vi "mac_mem_dot_product2.vi"() -> ()   [LabVIEW 2014]
uses:
  <vilib>/rvi/XilinxIP/XIPIN_XNode/niFpgaXIPIN.xnode
  <vilib>/Platform/TimedLoop/XDataNode/XDataNode.xnode
  <vilib>/Platform/TimedLoop/XDataNode/nitl_modes.ctl
  <vilib>/Platform/TimedLoop/XDataNode/XDNodeRunTimeDep.lvlib
  <vilib>/Platform/TimedLoop/XDataNode/wakeup.ctl
  <vilib>/Platform/TimedLoop/XDataNode/timing_clust.ctl
  <vilib>/rvi/DataTransferAndStorage/Container/XNode/niFpgaContainer.xnode
  <vilib>/rvi/IPIntegrationNode/IPINode_Xnode/niFpgaIPINode.xnode
  <vilib>/rvi/Memory/Memory_Emulation/niFpgaMemoryEmulationRefIn.vi
  afm_MPC_project/fpga_quadProg/mac_example/Multiply Accumulator12/Multiply_Accumulator12_8251C0362ABC46F4A5B5600C6E330BA5.dll
  MAC_project/mac_example/Multiply Accumulator 6 2 1 2/Multiply_Accumulator_6_2_1_2_02FD3C74846A4C02A23212CAACE05444.dll
  afm_MPC_project/fpga_quadProg/mac_example/Multiply Accumulator10/Multiply_Accumulator10_12FF9FB1410E45B083B4D52CE0C0E68A.dll
  afm_MPC_project/fpga_quadProg/mac_example/Multiply Accumulator09/Multiply_Accumulator09_5D60E3E552CB475F9C9DEB2CB9D60D9C.dll
  afm_MPC_project/fpga_quadProg/mac_example/Multiply Accumulator08/Multiply_Accumulator08_63B3B19177EB4E2C93FF5B78B22982AF.dll
  afm_MPC_project/fpga_quadProg/mac_example/Multiply Accumulator07/Multiply_Accumulator07_E764427B2AF0450BAE442029304CE909.dll
  afm_MPC_project/fpga_quadProg/mac_example/Multiply Accumulator05/Multiply_Accumulator05_30F34FE4A0744937816A99E0FF75C50A.dll
  afm_MPC_project/fpga_quadProg/mac_example/Multiply Accumulator04/Multiply_Accumulator04_4CB6AC15FF37476DBC15807E3D8215EA.dll
  afm_MPC_project/fpga_quadProg/mac_example/Multiply Accumulator03/Multiply_Accumulator03_801B681484E74D9B98E4BDB409AD9BD2.dll
  afm_MPC_project/fpga_quadProg/mac_example/Multiply Accumulator02/Multiply_Accumulator02_E9BD86879A6F4953AE28C6201495FEE1.dll
  afm_MPC_project/fpga_quadProg/mac_example/Multiply Accumulator01/Multiply_Accumulator01_75DB40A42D7149569D987152CB0D01C1.dll
  afm_MPC_project/fpga_quadProg/mac_example/Multiply Accumulator13/Multiply_Accumulator13_12AB7DA088AB48F383581A6BB4F5EF48.dll
  afm_MPC_project/fpga_quadProg/mac_example/Multiply Accumulator15/Multiply_Accumulator15_AA46839E45CE4F01941F3EA3B8C129F7.dll
  afm_MPC_project/fpga_quadProg/mac_example/Multiply Accumulator16/Multiply_Accumulator16_19D64967FE2446C38501744F7FD46696.dll
  afm_MPC_project/fpga_quadProg/mac_example/Multiply Accumulator17/Multiply_Accumulator17_68B37788AA734A29A986F77D953AD864.dll
  afm_MPC_project/fpga_quadProg/mac_example/Multiply Accumulator18/Multiply_Accumulator18_9000D848DA044E598463B90A0F5FDA52.dll
  afm_MPC_project/fpga_quadProg/mac_example/Multiply Accumulator19/Multiply_Accumulator19_D9569D38672A42FAB612A6C6146A7F7D.dll
  afm_MPC_project/fpga_quadProg/mac_example/Multiply Accumulator20/Multiply_Accumulator20_39D8BFFDA167413996EF3D9E83AB1150.dll
  afm_MPC_project/fpga_quadProg/mac_example/Multiply Accumulator21/Multiply_Accumulator21_1E0469235E034C438B32764042598187.dll
  afm_MPC_project/fpga_quadProg/mac_example/Multiply Accumulator22/Multiply_Accumulator22_BD44292DDFE84C49BBDF0A5781548576.dll
  afm_MPC_project/fpga_quadProg/mac_example/Multiply Accumulator23/Multiply_Accumulator23_14E7B3DBE11448D3B90B25377FD6EA57.dll
  afm_MPC_project/fpga_quadProg/mac_example/Multiply Accumulator24/Multiply_Accumulator24_B8B0017A331E415CA2A56A1A38052C9D.dll
  MAC_project/mac_example/Multiply Accumulator06 2/Multiply_Accumulator06_2_FA45EE958C1E4FC79E4A67AB6AD01B1E.dll
  afm_MPC_project/fpga_quadProg/mac_example/Multiply Accumulator14/Multiply_Accumulator14_5D647B84DE964E6297114951802A7EF8.dll
  <vilib>/rvi/IPIntegrationNode/IPINode_Typedef/niFpgaIPINodeSupportedFamilies.ctl
  <vilib>/rvi/IPIntegrationNode/IPINode_Utilities/niFpgaIPINodeSimCore.vi
panel:
  in  "Ns":i16
  out "appended array":fxp<+/-,32,7>[](array[numeric])
  out "s":fxp<+/-,32,7>
  in  "Array":fxp<+/-,18,5>[](array[numeric])=[0.0, 0.0, 0.0, 0.0, 0.0, 0.0, 0.0, 0.0, 0.0, 0.0, 0.0, 0.0, 0.0, 0.0, 0.0, 0.0, 0.0, 0.0, 0.0, 0.0, 0.0, 0.0, 0.0, 0.0]
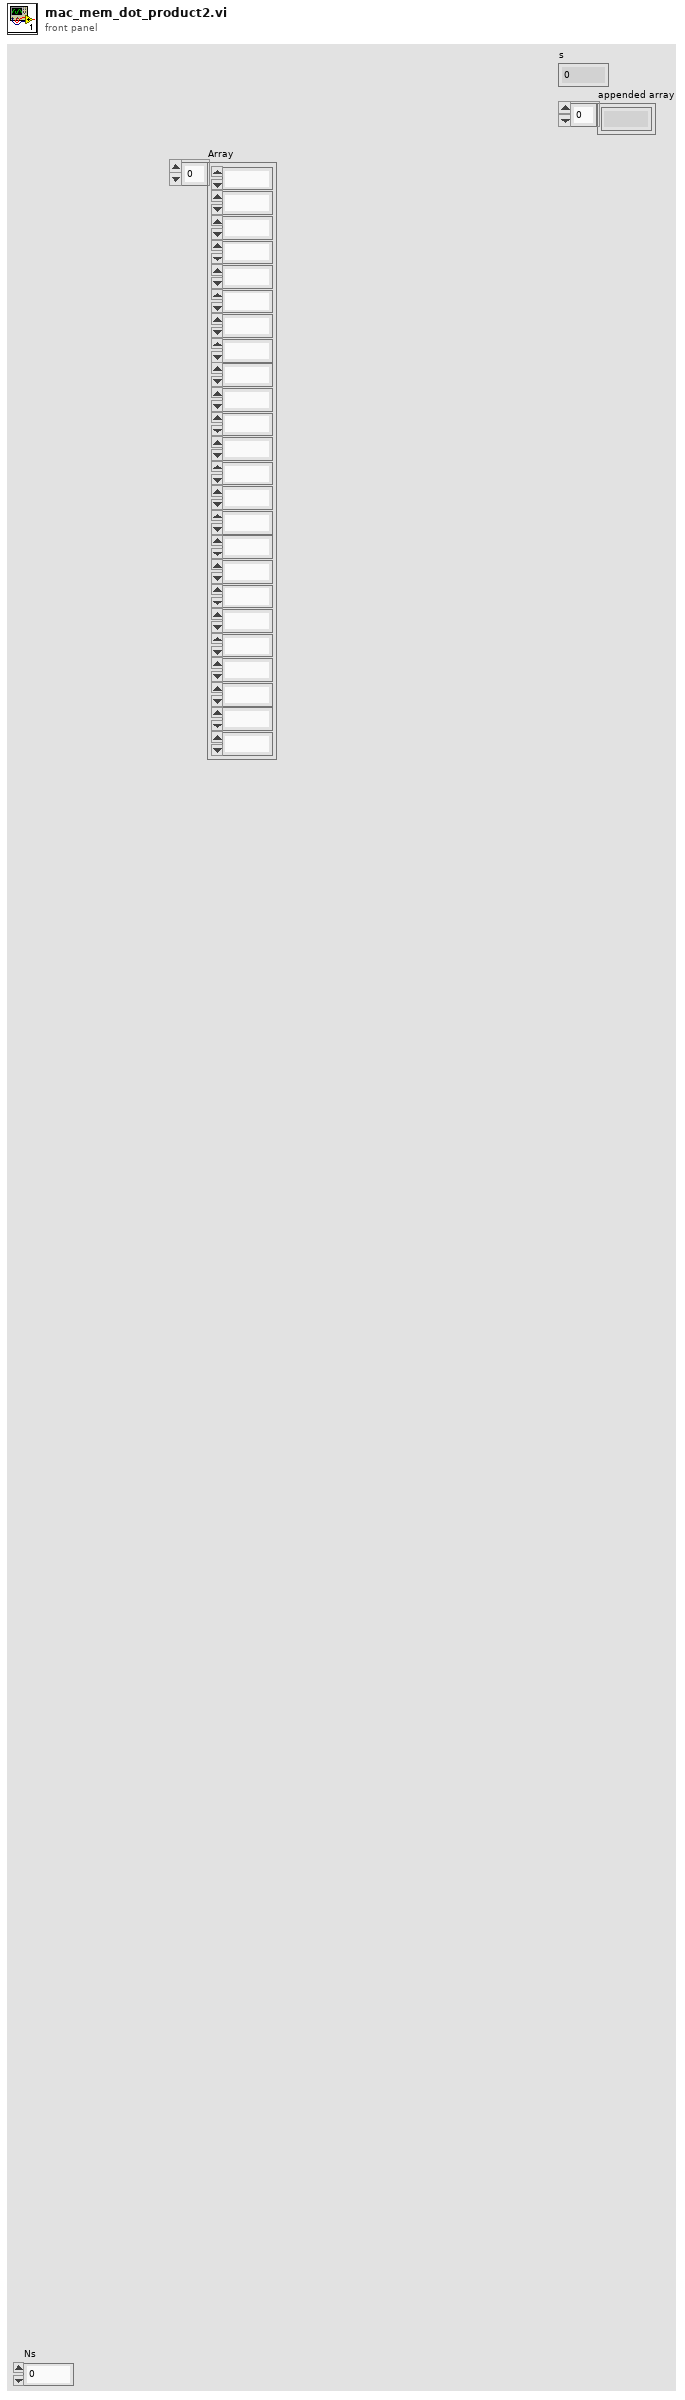
[diagram p1: front panel]
types:
  T1 = typedef "XDNodeRunTimeDep.lvlib/timing_clust.ctl" = cluster{"Expected End [f-1]":u64, "Actual End [f-1]":u64, "Finished Late? [f-1]":bool, "Expected End [i-1]":u64, "Actual End [i-1]":u64, "Finished Late? [i-1]":bool, "Expected Start [i]":u64, "Actual Start [i]":u64, "Expected Start [f]":u64, "Actual Start [f]":u64, "Source Name":string, "Structure Name":string, "Period":i64, "Deadline":i64, "Offset":i64, "Start":i64, "Priority":i32, "Timeout":i32, "Mode":T2, "Wakeup Reason":T3, "Error":errorcluster, "Source Type":string, "Secondary Source Type":string, "Global End Time":u64, "Global Start Time":u64, "Frame Duration":u64, "Iteration Duration":u64, "Assigned CPU":i32, "I/O Scan Engine Mode":u32}
  T2 = typedef "XDNodeRunTimeDep.lvlib/nitl_modes.ctl" = enum32{"No Change", "Process missed periods, maintain original phase", "Discard missed periods, maintain original phase", "Process missed periods, ignore original phase", "Discard missed periods, ignore original phase"}
  T3 = typedef "XDNodeRunTimeDep.lvlib/wakeup.ctl" = enum32{"Normal", "Aborted", "Asynchronous wakeup", "Timing source error", "Timed loop error", "Timeout"}
  T4 = typedef "niFpgaIPINodeSupportedFamilies.ctl" = cluster{"unlimited?":bool, "supported targets":string[]}
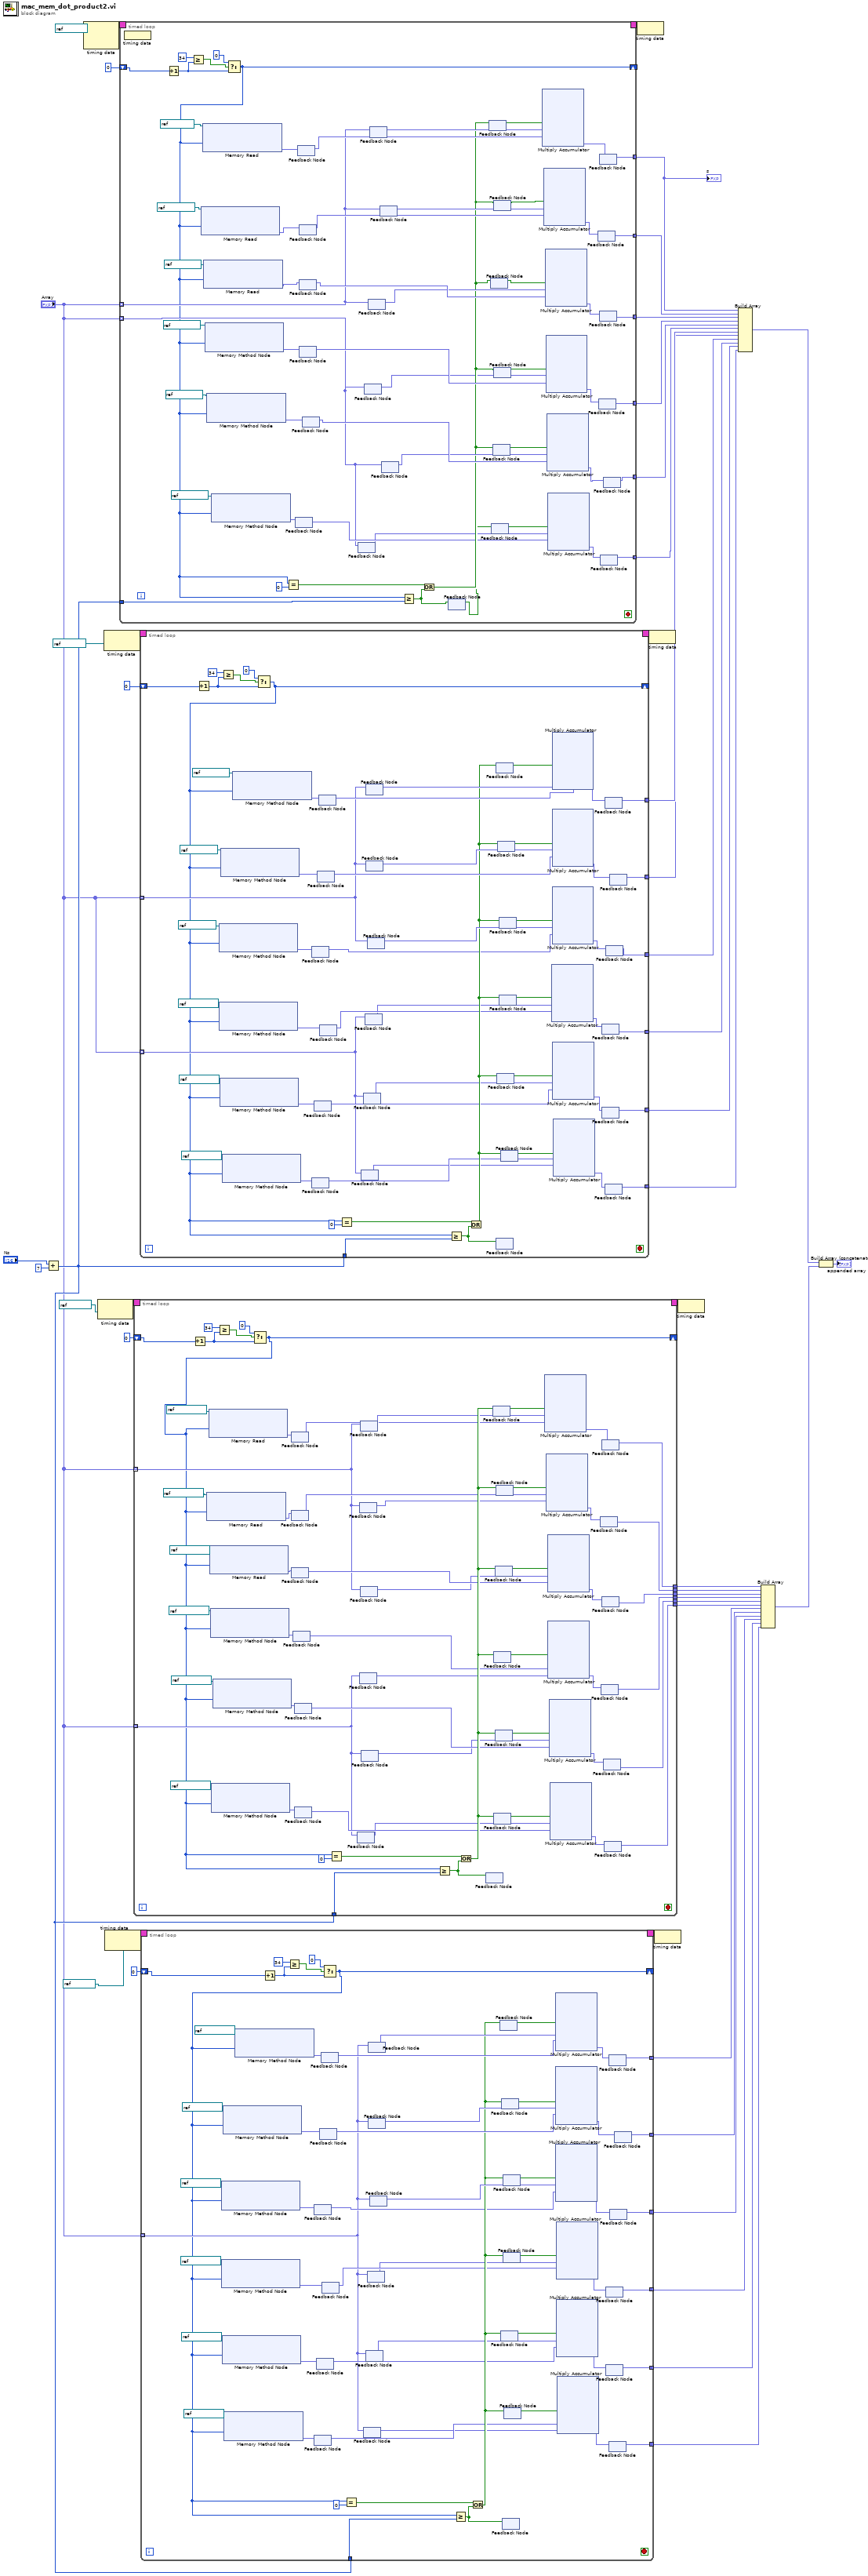
[diagram p0: block diagram]
diagram:
  n1 = Add(x="Ns", y=i16 7) -> (x+y=w8:i16)
  n2 = node-c288(refnum<k21> "160MHz" ("Source Name")) -> (w21:T1)  [unwired: 1 in]
  n3 = node-c288(refnum<k21> "160MHz" ("Source Name")) -> (w13:T1)
  n4 = node-c288(refnum<k21> "160MHz" ("Source Name")) -> (w19:T1)
  n5 = node-c288(refnum<k21> "160MHz" ("Source Name")) -> (w10:T1)
  n6 = timed-loop {
    timing: w21 -> [_]
    timing-out: [_] -> w20
    tunnel: [w103] -> w47
    tunnel: [w102] -> w46
    tunnel: [w101] -> w45
    tunnel: [w100] -> w44
    tunnel: [w99] -> w43
    tunnel: "Array" -> [w64] mode=indexing
    tunnel: w8 -> [w85]
    tunnel: "Array" -> [w56] mode=indexing
    tunnel: [w55] -> w6
    shift-right: [w48] -> _
    shift-left: i16 0 -> [w53]
    stop <- _ stop-if-true
    n7 = node-c288() -> ()  [unwired: 1 in]
    n8 = Increment(x=w53) -> (x+1=w52:i16)
    n9 = Greater Or Equal?(x=i16 34, y=w52) -> (x >= y?=w51:bool)
    n10 = Select(t=i16 0, s=w51, f=w52) -> (s? t:f=w48:i16)
    n11 = xnode ("Memory Read")("Address"=w48, "Memory In"=refnum<k21> "Memory 2") -> ("Data"=w80:fxp<+/-,32,2>)  [unwired: 1 out]
    n12 = xnode ("Memory Read")("Address"=w48, "Memory In"=refnum<k21> "Memory") -> ("Data"=w84:fxp<+/-,32,2>)  [unwired: 1 out]
    n13 = xnode ("Memory Read")("Address"=w48, "Memory In"=refnum<k21> "Memory 3") -> ("Data"=w77:fxp<+/-,32,2>)  [unwired: 1 out]
    n14 = xnode ("Memory Method Node")("Address"=w48, "Memory In"=refnum<k21> "Memory 4") -> ("Data"=w74:fxp<+/-,32,2>)  [unwired: 1 out]
    n15 = xnode ("Memory Method Node")("Address"=w48, "Memory In"=refnum<k21> "Memory 5") -> ("Data"=w72:fxp<+/-,32,2>)  [unwired: 1 out]
    n16 = xnode ("Memory Method Node")("Address"=w48, "Memory In"=refnum<k21> "Memory 6") -> ("Data"=w62:fxp<+/-,32,2>)  [unwired: 1 out]
    n17 = Equal?(x=w48, y=0) -> (x = y?=w86:bool)
    n18 = feedback #1() -> (w59:fxp<+/-,32,2>)  [unwired: 1 in]
    n19 = feedback-in #1(w62) -> ()
    n20 = feedback #2() -> (w83:fxp<+/-,32,2>)  [unwired: 1 in]
    n21 = feedback-in #2(w84) -> ()
    n22 = feedback #3() -> (w81:fxp<+/-,32,2>)  [unwired: 1 in]
    n23 = feedback-in #3(w80) -> ()
    n24 = feedback #4() -> (w78:fxp<+/-,32,2>)  [unwired: 1 in]
    n25 = feedback-in #4(w77) -> ()
    n26 = feedback #5() -> (w75:fxp<+/-,32,2>)  [unwired: 1 in]
    n27 = feedback-in #5(w74) -> ()
    n28 = feedback #6() -> (w73:fxp<+/-,32,2>)  [unwired: 1 in]
    n29 = feedback-in #6(w72) -> ()
    n30 = feedback #7() -> (w58:fxp<+/-,18,5>)  [unwired: 1 in]
    n31 = feedback-in #7(w56) -> ()
    n32 = feedback #8() -> (w54:fxp<+/-,18,5>)  [unwired: 1 in]
    n33 = feedback-in #8(w56) -> ()
    n34 = feedback #9() -> (w76:fxp<+/-,18,5>)  [unwired: 1 in]
    n35 = feedback-in #9(w64) -> ()
    n36 = feedback #10() -> (w82:fxp<+/-,18,5>)  [unwired: 1 in]
    n37 = feedback-in #10(w64) -> ()
    n38 = feedback #11() -> (w79:fxp<+/-,18,5>)  [unwired: 1 in]
    n39 = feedback-in #11(w64) -> ()
    n40 = feedback #12() -> (w71:fxp<+/-,18,5>)  [unwired: 1 in]
    n41 = feedback-in #12(w56) -> ()
    n42 = Greater Or Equal?(x=w48, y=w85) -> (x >= y?=w70:bool)
    n43 = Or(x=w86, y=w70) -> (x .or. y?=w66:bool)
    n44 = feedback #13() -> (w57:bool)  [unwired: 1 in]
    n45 = feedback-in #13(w70) -> ()
    n46 = feedback #14() -> (w65:bool)  [unwired: 1 in]
    n47 = feedback-in #14(w66) -> ()
    n48 = feedback #15() -> (w68:bool)  [unwired: 1 in]
    n49 = feedback-in #15(w66) -> ()
    n50 = feedback #16() -> (w61:bool)  [unwired: 1 in]
    n51 = feedback-in #16(w57) -> ()
    n52 = feedback #17() -> (w93:bool)  [unwired: 1 in]
    n53 = feedback-in #17(w66) -> ()
    n54 = feedback #18() -> (w69:bool)  [unwired: 1 in]
    n55 = feedback-in #18(w66) -> ()
    n56 = feedback #19() -> (w67:bool)  [unwired: 1 in]
    n57 = feedback-in #19(w66) -> ()
    n58 = xnode ("Multiply Accumulator")("sclr"=w65, "b"=w82, "a"=w83) -> ("s"=w88:fxp<+/-,32,7>)  [unwired: 2 in]
    n59 = xnode ("Multiply Accumulator")("sclr"=w67, "b"=w79, "a"=w81) -> ("s"=w89:fxp<+/-,32,7>)  [unwired: 2 in]
    n60 = xnode ("Multiply Accumulator")("sclr"=w68, "b"=w76, "a"=w78) -> ("s"=w90:fxp<+/-,32,7>)  [unwired: 2 in]
    n61 = xnode ("Multiply Accumulator")("sclr"=w69, "b"=w54, "a"=w75) -> ("s"=w91:fxp<+/-,32,7>)  [unwired: 2 in]
    n62 = xnode ("Multiply Accumulator")("sclr"=w93, "b"=w71, "a"=w73) -> ("s"=w92:fxp<+/-,18,7>)  [unwired: 2 in]
    n63 = xnode ("Multiply Accumulator")("sclr"=w61, "b"=w58, "a"=w59) -> ("s"=w60:fxp<+/-,32,7>)  [unwired: 2 in]
    n64 = feedback #20() -> (w102:fxp<+/-,32,7>)  [unwired: 1 in]
    n65 = feedback-in #20(w89) -> ()
    n66 = feedback #21() -> (w100:fxp<+/-,32,7>)  [unwired: 1 in]
    n67 = feedback-in #21(w91) -> ()
    n68 = feedback #22() -> (w103:fxp<+/-,32,7>)  [unwired: 1 in]
    n69 = feedback-in #22(w88) -> ()
    n70 = feedback #23() -> (w101:fxp<+/-,32,7>)  [unwired: 1 in]
    n71 = feedback-in #23(w90) -> ()
    n72 = feedback #24() -> (w55:fxp<+/-,32,7>)  [unwired: 1 in]
    n73 = feedback-in #24(w60) -> ()
    n74 = feedback #25() -> (w99:fxp<+/-,18,7>)  [unwired: 1 in]
    n75 = feedback-in #25(w92) -> ()
  }
  "s" <- w47
  n76 = timed-loop {
    timing: w13 -> [_]
    timing-out: [_] -> w12
    tunnel: [w439] -> w36
    tunnel: [w438] -> w35
    tunnel: [w437] -> w34
    tunnel: [w436] -> w33
    tunnel: [w435] -> w32
    tunnel: [w434] -> w31
    tunnel: "Array" -> [w392] mode=indexing
    tunnel: w8 -> [w406]
    tunnel: "Array" -> [w391] mode=indexing
    shift-right: [w385] -> _
    shift-left: i16 0 ("t") -> [w386]
    stop <- _ stop-if-true
    n77 = Increment(x=w386) -> (x+1=w390:i16)
    n78 = Greater Or Equal?(x=i16 34, y=w390) -> (x >= y?=w389:bool)
    n79 = Select(t=i16 0, s=w389, f=w390) -> (s? t:f=w385:i16)
    n80 = xnode ("Memory Read")("Address"=w385, "Memory In"=refnum<k21> "Memory 14") -> ("Data"=w431:fxp<+/-,32,2>)  [unwired: 1 out]
    n81 = xnode ("Memory Read")("Address"=w385, "Memory In"=refnum<k21> "Memory 13") -> ("Data"=w430:fxp<+/-,32,2>)  [unwired: 1 out]
    n82 = xnode ("Memory Read")("Address"=w385, "Memory In"=refnum<k21> "Memory 15") -> ("Data"=w428:fxp<+/-,32,2>)  [unwired: 1 out]
    n83 = xnode ("Memory Method Node")("Address"=w385, "Memory In"=refnum<k21> "Memory 16") -> ("Data"=w426:fxp<+/-,32,2>)  [unwired: 1 out]
    n84 = xnode ("Memory Method Node")("Address"=w385, "Memory In"=refnum<k21> "Memory 18") -> ("Data"=w422:fxp<+/-,32,2>)  [unwired: 1 out]
    n85 = xnode ("Memory Method Node")("Address"=w385, "Memory In"=refnum<k21> "Memory 17") -> ("Data"=w424:fxp<+/-,32,2>)  [unwired: 1 out]
    n86 = feedback #26() -> (w401:fxp<+/-,32,2>)  [unwired: 1 in]
    n87 = feedback-in #26(w431) -> ()
    n88 = feedback #27() -> (w403:fxp<+/-,32,2>)  [unwired: 1 in]
    n89 = feedback-in #27(w430) -> ()
    n90 = feedback #28() -> (w400:fxp<+/-,32,2>)  [unwired: 1 in]
    n91 = feedback-in #28(w428) -> ()
    n92 = feedback #29() -> (w398:fxp<+/-,32,2>)  [unwired: 1 in]
    n93 = feedback-in #29(w426) -> ()
    n94 = feedback #30() -> (w396:fxp<+/-,32,2>)  [unwired: 1 in]
    n95 = feedback-in #30(w424) -> ()
    n96 = feedback #31() -> (w394:fxp<+/-,32,2>)  [unwired: 1 in]
    n97 = feedback-in #31(w422) -> ()
    n98 = Equal?(x=w385, y=0) -> (x = y?=w408:bool)
    n99 = feedback #32() -> (w393:fxp<+/-,18,5>)  [unwired: 1 in]
    n100 = feedback-in #32(w391) -> ()
    n101 = feedback #33() -> (w402:fxp<+/-,18,5>)  [unwired: 1 in]
    n102 = feedback-in #33(w392) -> ()
    n103 = feedback #34() -> (w397:fxp<+/-,18,5>)  [unwired: 1 in]
    n104 = feedback-in #34(w391) -> ()
    n105 = feedback #35() -> (w404:fxp<+/-,18,5>)  [unwired: 1 in]
    n106 = feedback-in #35(w392) -> ()
    n107 = feedback #36() -> (w399:fxp<+/-,18,5>)  [unwired: 1 in]
    n108 = feedback-in #36(w392) -> ()
    n109 = feedback #37() -> (w395:fxp<+/-,18,5>)  [unwired: 1 in]
    n110 = feedback-in #37(w391) -> ()
    n111 = Greater Or Equal?(x=w385, y=w406) -> (x >= y?=w407:bool)
    n112 = Or(x=w408, y=w407) -> (x .or. y?=w405:bool)
    n113 = feedback #38() -> ()  [unwired: 2 in]
    n114 = feedback-in #38(w407) -> ()
    n115 = feedback #39() -> (w416:bool)  [unwired: 1 in]
    n116 = feedback-in #39(w405) -> ()
    n117 = feedback #40() -> (w419:bool)  [unwired: 1 in]
    n118 = feedback-in #40(w405) -> ()
    n119 = feedback #41() -> (w421:bool)  [unwired: 1 in]
    n120 = feedback-in #41(w405) -> ()
    n121 = feedback #42() -> (w418:bool)  [unwired: 1 in]
    n122 = feedback-in #42(w405) -> ()
    n123 = feedback #43() -> (w420:bool)  [unwired: 1 in]
    n124 = feedback-in #43(w405) -> ()
    n125 = feedback #44() -> (w417:bool)  [unwired: 1 in]
    n126 = feedback-in #44(w405) -> ()
    n127 = xnode ("Multiply Accumulator")("sclr"=w416, "b"=w404, "a"=w403) -> ("s"=w410:fxp<+/-,32,7>)  [unwired: 2 in]
    n128 = xnode ("Multiply Accumulator")("sclr"=w417, "a"=w401, "b"=w402) -> ("s"=w411:fxp<+,16,16>)  [unwired: 2 in]
    n129 = xnode ("Multiply Accumulator")("sclr"=w418, "b"=w399, "a"=w400) -> ("s"=w412:fxp<+/-,32,7>)  [unwired: 2 in]
    n130 = xnode ("Multiply Accumulator")("sclr"=w419, "b"=w397, "a"=w398) -> ("s"=w413:fxp<+/-,32,7>)  [unwired: 2 in]
    n131 = xnode ("Multiply Accumulator")("sclr"=w420, "b"=w395, "a"=w396) -> ("s"=w414:fxp<+/-,32,7>)  [unwired: 2 in]
    n132 = xnode ("Multiply Accumulator")("sclr"=w421, "b"=w393, "a"=w394) -> ("s"=w415:fxp<+/-,32,7>)  [unwired: 2 in]
    n133 = feedback #45() -> (w438:fxp<+,16,16>)  [unwired: 1 in]
    n134 = feedback-in #45(w411) -> ()
    n135 = feedback #46() -> (w436:fxp<+/-,32,7>)  [unwired: 1 in]
    n136 = feedback-in #46(w413) -> ()
    n137 = feedback #47() -> (w439:fxp<+/-,32,7>)  [unwired: 1 in]
    n138 = feedback-in #47(w410) -> ()
    n139 = feedback #48() -> (w437:fxp<+/-,32,7>)  [unwired: 1 in]
    n140 = feedback-in #48(w412) -> ()
    n141 = feedback #49() -> (w435:fxp<+/-,32,7>)  [unwired: 1 in]
    n142 = feedback-in #49(w414) -> ()
    n143 = feedback #50() -> (w434:fxp<+/-,32,7>)  [unwired: 1 in]
    n144 = feedback-in #50(w415) -> ()
  }
  n145 = timed-loop {
    timing: w19 -> [_]
    timing-out: [_] -> w18
    tunnel: w8 -> [w826]
    tunnel: [w825] -> w42
    tunnel: [w824] -> w41
    tunnel: [w823] -> w40
    tunnel: [w822] -> w39
    tunnel: [w821] -> w38
    tunnel: [w820] -> w37
    tunnel: "Array" -> [w779] mode=indexing
    tunnel: "Array" -> [w778] mode=indexing
    shift-right: [w772] -> _
    shift-left: i16 0 ("t") -> [w773]
    stop <- _ stop-if-true
    n146 = Increment(x=w773) -> (x+1=w777:i16)
    n147 = Greater Or Equal?(x=i16 34, y=w777) -> (x >= y?=w776:bool)
    n148 = Select(t=i16 0, s=w776, f=w777) -> (s? t:f=w772:i16)
    n149 = xnode ("Memory Method Node")("Address"=w772, "Memory In"=refnum<k21> "Memory 9") -> ("Data"=w794:fxp<+/-,32,2>)  [unwired: 1 out]
    n150 = xnode ("Memory Method Node")("Address"=w772, "Memory In"=refnum<k21> "Memory 10") -> ("Data"=w795:fxp<+/-,32,2>)  [unwired: 1 out]
    n151 = xnode ("Memory Method Node")("Address"=w772, "Memory In"=refnum<k21> "Memory 11") -> ("Data"=w796:fxp<+/-,32,2>)  [unwired: 1 out]
    n152 = xnode ("Memory Method Node")("Address"=w772, "Memory In"=refnum<k21> "Memory 8") -> ("Data"=w808:fxp<+/-,32,2>)  [unwired: 1 out]
    n153 = xnode ("Memory Method Node")("Address"=w772, "Memory In"=refnum<k21> "Memory 12") -> ("Data"=w797:fxp<+/-,32,2>)  [unwired: 1 out]
    n154 = xnode ("Memory Method Node")("Address"=w772, "Memory In"=refnum<k21> "Memory 7") -> ("Data"=w806:fxp<+/-,32,2>)  [unwired: 1 out]
    n155 = feedback #51() -> (w793:fxp<+/-,32,2>)  [unwired: 1 in]
    n156 = feedback-in #51(w794) -> ()
    n157 = feedback #52() -> (w790:fxp<+/-,32,2>)  [unwired: 1 in]
    n158 = feedback-in #52(w797) -> ()
    n159 = feedback #53() -> (w791:fxp<+/-,32,2>)  [unwired: 1 in]
    n160 = feedback-in #53(w796) -> ()
    n161 = feedback #54() -> (w807:fxp<+/-,32,2>)  [unwired: 1 in]
    n162 = feedback-in #54(w808) -> ()
    n163 = feedback #55() -> (w805:fxp<+/-,32,2>)  [unwired: 1 in]
    n164 = feedback-in #55(w806) -> ()
    n165 = feedback #56() -> (w792:fxp<+/-,32,2>)  [unwired: 1 in]
    n166 = feedback-in #56(w795) -> ()
    n167 = Equal?(x=w772, y=0) -> (x = y?=w818:bool)
    n168 = feedback #57() -> (w787:fxp<+/-,18,5>)  [unwired: 1 in]
    n169 = feedback-in #57(w778) -> ()
    n170 = feedback #58() -> (w788:fxp<+/-,18,5>)  [unwired: 1 in]
    n171 = feedback-in #58(w778) -> ()
    n172 = feedback #59() -> (w789:fxp<+/-,18,5>)  [unwired: 1 in]
    n173 = feedback-in #59(w778) -> ()
    n174 = feedback #60() -> (w814:fxp<+/-,18,5>)  [unwired: 1 in]
    n175 = feedback-in #60(w779) -> ()
    n176 = feedback #61() -> (w813:fxp<+/-,18,5>)  [unwired: 1 in]
    n177 = feedback-in #61(w779) -> ()
    n178 = feedback #62() -> (w812:fxp<+/-,18,5>)  [unwired: 1 in]
    n179 = feedback-in #62(w779) -> ()
    n180 = Greater Or Equal?(x=w772, y=w826) -> (x >= y?=w780:bool)
    n181 = Or(x=w818, y=w780) -> (x .or. y?=w799:bool)
    n182 = feedback #63() -> (w817:bool)  [unwired: 1 in]
    n183 = feedback-in #63(w799) -> ()
    n184 = feedback #64() -> ()  [unwired: 2 in]
    n185 = feedback-in #64(w780) -> ()
    n186 = feedback #65() -> (w800:bool)  [unwired: 1 in]
    n187 = feedback-in #65(w799) -> ()
    n188 = feedback #66() -> (w816:bool)  [unwired: 1 in]
    n189 = feedback-in #66(w799) -> ()
    n190 = feedback #67() -> (w815:bool)  [unwired: 1 in]
    n191 = feedback-in #67(w799) -> ()
    n192 = feedback #68() -> (w801:bool)  [unwired: 1 in]
    n193 = feedback-in #68(w799) -> ()
    n194 = feedback #69() -> (w798:bool)  [unwired: 1 in]
    n195 = feedback-in #69(w799) -> ()
    n196 = xnode ("Multiply Accumulator")("sclr"=w801, "b"=w789, "a"=w792) -> ("s"=w781:fxp<+/-,32,7>)  [unwired: 2 in]
    n197 = xnode ("Multiply Accumulator")("sclr"=w817, "b"=w814, "a"=w805) -> ("s"=w783:fxp<+/-,32,7>)  [unwired: 2 in]
    n198 = xnode ("Multiply Accumulator")("sclr"=w816, "b"=w813, "a"=w807) -> ("s"=w786:fxp<+/-,32,7>)  [unwired: 2 in]
    n199 = xnode ("Multiply Accumulator")("sclr"=w815, "b"=w812, "a"=w793) -> ("s"=w782:fxp<+/-,32,7>)  [unwired: 2 in]
    n200 = xnode ("Multiply Accumulator")("sclr"=w800, "b"=w788, "a"=w791) -> ("s"=w785:fxp<+/-,32,7>)  [unwired: 2 in]
    n201 = xnode ("Multiply Accumulator")("sclr"=w798, "b"=w787, "a"=w790) -> ("s"=w784:fxp<+/-,32,7>)  [unwired: 2 in]
    n202 = feedback #70() -> (w822:fxp<+/-,32,7>)  [unwired: 1 in]
    n203 = feedback-in #70(w781) -> ()
    n204 = feedback #71() -> (w821:fxp<+/-,32,7>)  [unwired: 1 in]
    n205 = feedback-in #71(w785) -> ()
    n206 = feedback #72() -> (w825:fxp<+/-,32,7>)  [unwired: 1 in]
    n207 = feedback-in #72(w783) -> ()
    n208 = feedback #73() -> (w820:fxp<+/-,32,7>)  [unwired: 1 in]
    n209 = feedback-in #73(w784) -> ()
    n210 = feedback #74() -> (w823:fxp<+/-,32,7>)  [unwired: 1 in]
    n211 = feedback-in #74(w782) -> ()
    n212 = feedback #75() -> (w824:fxp<+/-,32,7>)  [unwired: 1 in]
    n213 = feedback-in #75(w786) -> ()
  }
  n214 = timed-loop {
    timing: w10 -> [_]
    timing-out: [_] -> w9
    tunnel: [w1161] -> w30
    tunnel: [w1160] -> w29
    tunnel: [w1159] -> w28
    tunnel: [w1158] -> w27
    tunnel: [w1157] -> w26
    tunnel: [w1156] -> w25
    tunnel: w8 -> [w1155]
    tunnel: "Array" -> [w1114] mode=indexing
    shift-right: [w1108] -> _
    shift-left: i16 0 ("t") -> [w1109]
    stop <- _ stop-if-true
    n215 = Increment(x=w1109) -> (x+1=w1113:i16)
    n216 = Greater Or Equal?(x=i16 34, y=w1113) -> (x >= y?=w1112:bool)
    n217 = feedback #76() -> (w1128:fxp<+/-,32,2>)  [unwired: 1 in]
    n218 = feedback #77() -> (w1125:fxp<+/-,32,2>)  [unwired: 1 in]
    n219 = feedback #78() -> (w1126:fxp<+/-,32,2>)  [unwired: 1 in]
    n220 = feedback #79() -> (w1142:fxp<+/-,32,2>)  [unwired: 1 in]
    n221 = feedback #80() -> (w1140:fxp<+/-,32,2>)  [unwired: 1 in]
    n222 = feedback #81() -> (w1127:fxp<+/-,32,2>)  [unwired: 1 in]
    n223 = Select(t=i16 0, s=w1112, f=w1113) -> (s? t:f=w1108:i16)
    n224 = xnode ("Memory Method Node")("Address"=w1108, "Memory In"=refnum<k21> "Memory 21") -> ("Data"=w1129:fxp<+/-,32,2>)  [unwired: 1 out]
    n225 = xnode ("Memory Method Node")("Address"=w1108, "Memory In"=refnum<k21> "Memory 22") -> ("Data"=w1130:fxp<+/-,32,2>)  [unwired: 1 out]
    n226 = xnode ("Memory Method Node")("Address"=w1108, "Memory In"=refnum<k21> "Memory 23") -> ("Data"=w1131:fxp<+/-,32,2>)  [unwired: 1 out]
    n227 = xnode ("Memory Method Node")("Address"=w1108, "Memory In"=refnum<k21> "Memory 20") -> ("Data"=w1143:fxp<+/-,32,2>)  [unwired: 1 out]
    n228 = xnode ("Memory Method Node")("Address"=w1108, "Memory In"=refnum<k21> "Memory 24") -> ("Data"=w1132:fxp<+/-,32,2>)  [unwired: 1 out]
    n229 = xnode ("Memory Method Node")("Address"=w1108, "Memory In"=refnum<k21> "Memory 19") -> ("Data"=w1141:fxp<+/-,32,2>)  [unwired: 1 out]
    n230 = feedback-in #76(w1129) -> ()
    n231 = feedback-in #77(w1132) -> ()
    n232 = feedback-in #78(w1131) -> ()
    n233 = feedback-in #79(w1143) -> ()
    n234 = feedback-in #80(w1141) -> ()
    n235 = feedback-in #81(w1130) -> ()
    n236 = Equal?(x=w1108, y=0) -> (x = y?=w1153:bool)
    n237 = feedback #82() -> (w1122:fxp<+/-,18,5>)  [unwired: 1 in]
    n238 = feedback-in #82(w1114) -> ()
    n239 = feedback #83() -> (w1123:fxp<+/-,18,5>)  [unwired: 1 in]
    n240 = feedback-in #83(w1114) -> ()
    n241 = feedback #84() -> (w1124:fxp<+/-,18,5>)  [unwired: 1 in]
    n242 = feedback-in #84(w1114) -> ()
    n243 = feedback #85() -> (w1149:fxp<+/-,18,5>)  [unwired: 1 in]
    n244 = feedback-in #85(w1114) -> ()
    n245 = feedback #86() -> (w1148:fxp<+/-,18,5>)  [unwired: 1 in]
    n246 = feedback-in #86(w1114) -> ()
    n247 = feedback #87() -> (w1147:fxp<+/-,18,5>)  [unwired: 1 in]
    n248 = feedback-in #87(w1114) -> ()
    n249 = Greater Or Equal?(x=w1108, y=w1155) -> (x >= y?=w1115:bool)
    n250 = Or(x=w1153, y=w1115) -> (x .or. y?=w1134:bool)
    n251 = feedback #88() -> (w1152:bool)  [unwired: 1 in]
    n252 = feedback-in #88(w1134) -> ()
    n253 = feedback #89() -> (w1135:bool)  [unwired: 1 in]
    n254 = feedback-in #89(w1134) -> ()
    n255 = feedback #90() -> (w1151:bool)  [unwired: 1 in]
    n256 = feedback-in #90(w1134) -> ()
    n257 = feedback #91() -> ()  [unwired: 2 in]
    n258 = feedback-in #91(w1115) -> ()
    n259 = feedback #92() -> (w1150:bool)  [unwired: 1 in]
    n260 = feedback-in #92(w1134) -> ()
    n261 = feedback #93() -> (w1136:bool)  [unwired: 1 in]
    n262 = feedback-in #93(w1134) -> ()
    n263 = feedback #94() -> (w1133:bool)  [unwired: 1 in]
    n264 = feedback-in #94(w1134) -> ()
    n265 = xnode ("Multiply Accumulator")("sclr"=w1152, "b"=w1149, "a"=w1140) -> ("s"=w1118:fxp<+/-,32,7>)  [unwired: 2 in]
    n266 = xnode ("Multiply Accumulator")("sclr"=w1151, "b"=w1148, "a"=w1142) -> ("s"=w1121:fxp<+/-,32,7>)  [unwired: 2 in]
    n267 = xnode ("Multiply Accumulator")("sclr"=w1150, "b"=w1147, "a"=w1128) -> ("s"=w1117:fxp<+/-,32,7>)  [unwired: 2 in]
    n268 = xnode ("Multiply Accumulator")("sclr"=w1136, "b"=w1124, "a"=w1127) -> ("s"=w1116:fxp<+/-,32,7>)  [unwired: 2 in]
    n269 = xnode ("Multiply Accumulator")("sclr"=w1135, "b"=w1123, "a"=w1126) -> ("s"=w1120:fxp<+/-,32,7>)  [unwired: 2 in]
    n270 = xnode ("Multiply Accumulator")("sclr"=w1133, "b"=w1122, "a"=w1125) -> ("s"=w1119:fxp<+/-,32,7>)  [unwired: 2 in]
    n271 = feedback #95() -> (w1158:fxp<+/-,32,7>)  [unwired: 1 in]
    n272 = feedback-in #95(w1116) -> ()
    n273 = feedback #96() -> (w1157:fxp<+/-,32,7>)  [unwired: 1 in]
    n274 = feedback-in #96(w1120) -> ()
    n275 = feedback #97() -> (w1161:fxp<+/-,32,7>)  [unwired: 1 in]
    n276 = feedback-in #97(w1118) -> ()
    n277 = feedback #98() -> (w1156:fxp<+/-,32,7>)  [unwired: 1 in]
    n278 = feedback-in #98(w1119) -> ()
    n279 = feedback #99() -> (w1159:fxp<+/-,32,7>)  [unwired: 1 in]
    n280 = feedback-in #99(w1117) -> ()
    n281 = feedback #100() -> (w1160:fxp<+/-,32,7>)  [unwired: 1 in]
    n282 = feedback-in #100(w1121) -> ()
  }
  n283 = node-c288(w20) -> ()
  n284 = node-c288(w18) -> ()
  n285 = node-c288(w9) -> ()
  n286 = node-c288(w12) -> ()
  n287 = Build Array(w47, w46, w45, w44, w43, w6, w42, w41, w40, w39, w38, w37) -> (w24:fxp<+/-,32,7>[])
  n288 = Build Array(w36, w35, w34, w33, w32, w31, w30, w29, w28, w27, w26, w25) -> (w23:fxp<+/-,42,17>[])
  n289 = Build Array (concatenate)(w24, w23) -> (→"appended array":fxp<+/-,42,17>[])
